vi "DHE_GetobsID.vi"(8 "error in (no error)":errorcluster) -> (0 "error out":errorcluster, 2 "obsID":string)   [LabVIEW 2016]
uses:
  DBSHAND/private/vis/DatabaseHand_Element_Get(bool).vi
  DBSHAND/private/vis/DatabaseHand_Element_Get(string).vi
  DBSHAND/private/vis/DatabaseHand_Element_Get(U32).vi
  DBSHAND/private/vis/DatabaseHand_Element_Set(string).vi
  DBSHAND/private/vis/DatabaseHand_Element_Set(U32).vi
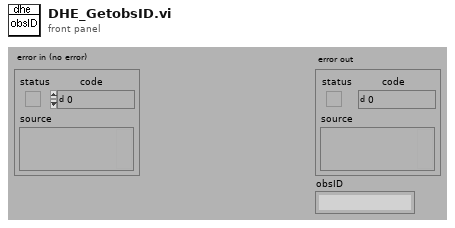
[diagram p1: front panel]
types:
  T1 = typedef "DatabaseHand_RefNum.ctl" = refnum<vi>
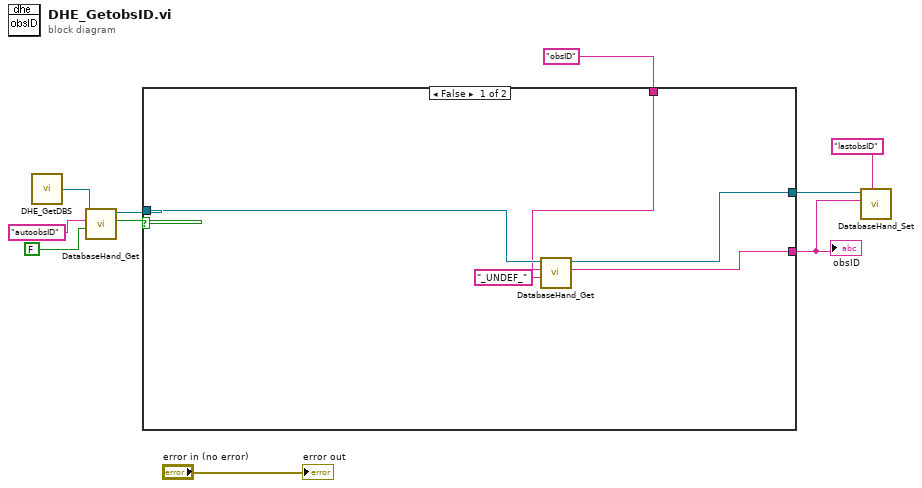
[diagram p0: block diagram]
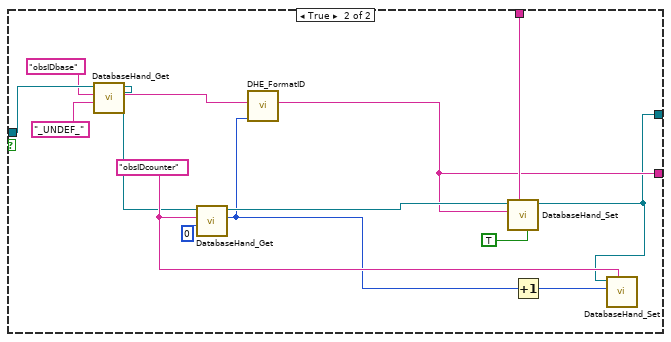
[diagram p2: hidden frame]
diagram:
  n1 = call "DHE_GetDBS.vi"() -> ("DHE_DBSRef"=w10:T1)  [unwired: 9 out]
  n2 = call-poly "DatabaseHand_Get.vi"("default value"=FALSE, "name"="autoobsID", "Database RefNum in"=w10) -> ("value"=w7:bool, "Database RefNum out"=w6:T1)  [unwired: 2 in, 5 out]
  n3 = case shown="False" w7 {
    tunnel: w6 -> [w15 w29]
    tunnel: [w13 w17] -> w2
    tunnel: "obsID" ("name") -> [w14 w21]
    tunnel: [w12 w16] -> w1
    frame False {
      n4 = call-poly "DatabaseHand_Get.vi"("default value"="_UNDEF_", "name"=w14, "Database RefNum in"=w15) -> ("value"=w13:string, "Database RefNum out"=w12:T1)  [unwired: 2 in, 5 out]
    }
    frame True {
      w24 = "obsIDcounter" ("name")
      n5 = call-poly "DatabaseHand_Get.vi"("default value"="_UNDEF_", "name"="obsIDbase", "Database RefNum in"=w29) -> ("value"=w20:string, "Database RefNum out"=w22:T1)  [unwired: 2 in, 5 out]
      n6 = call-poly "DatabaseHand_Get.vi"("default value"=u32 0 ("input 1"), "name"=w24, "Database RefNum in"=w22) -> ("value"=w19:u32, "Database RefNum out"=w26:T1)  [unwired: 2 in, 5 out]
      n7 = call "DHE_FormatID.vi"("id counter in"=w19, "IDbase in"=w20) -> ("expID out"=w17:string)  [unwired: 1 in, 8 out]
      n8 = call-poly "DatabaseHand_Set.vi"("enqueue? (F)"=TRUE, "name"=w21, "value"=w17, "Database RefNum in"=w26) -> ("Database RefNum out"=w16:T1)  [unwired: 4 in, 3 out]
      n9 = Increment(x=w19) -> (x+1=w23:u32)
      n10 = call-poly "DatabaseHand_Set.vi"("name"=w24, "value"=w23, "Database RefNum in"=w16) -> ()  [unwired: 5 in, 4 out]
    }
  }
  "obsID" <- w2
  n11 = call-poly "DatabaseHand_Set.vi"("name"="lastobsID", "value"=w2, "Database RefNum in"=w1) -> ()  [unwired: 5 in, 4 out]
  "error out" <- "error in (no error)"
